vi "GetHWDeviceName.vi"(8 "Error In":errorcluster, 11 "object in":refnum<class "Hardware.lvclass">) -> (0 "Error Out":errorcluster, 2 "HW Device Name":string, 3 "object out":refnum<class "Hardware.lvclass">)   [LabVIEW 2023, in "HAL.lvlib" / "Hardware.lvclass"]
uses:
  Hardware.lvclass
  Hardware.lvclass/Hardware.ctl
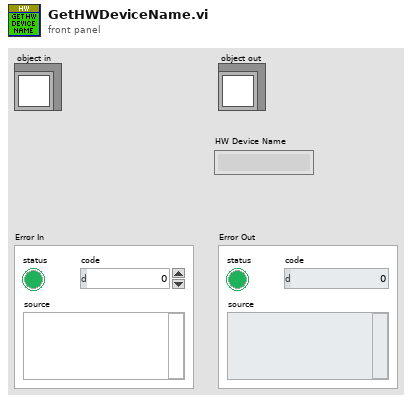
[diagram p1: front panel]
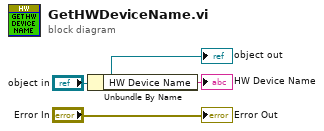
[diagram p0: block diagram]
diagram:
  n1 = Unbundle By Name("object in") -> ("HW Device Name"=→"HW Device Name":string)
  "Error Out" <- "Error In"
  "object out" <- "object in"
